vi "Inverse_Kinematics_noErrMsg_v1.vi"(4 "B3":dbl[](array[numeric]), 5 "px":dbl, 6 "pz":dbl, 7 "B2":dbl[](array[numeric]), 8 "py":dbl, 9 "B1":dbl[](array[numeric])) -> (1 "theta 3":sgl, 2 "theta 2":sgl, 3 "theta 1":sgl)   [LabVIEW 2010]
doc: "This VI converts the desired tool tip position (px,py,pz) into joint motions of theta 1, theta 2, and theta 3.\nB1, B2, and B3 are 2-element arrays containing lower and upper bounds for joint motions.\n\"Reset Inputs\" sends out a boolean value (T) if an error occurs."
panel:
  out "theta 3 LB":dbl
  out "theta 3 UB":dbl
  out "theta 2 LB":dbl
  out "theta 2 UB":dbl
  out "theta 1 LB":dbl
  out "theta 1 UB":dbl
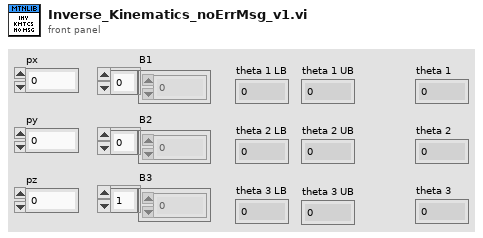
[diagram p1: front panel]
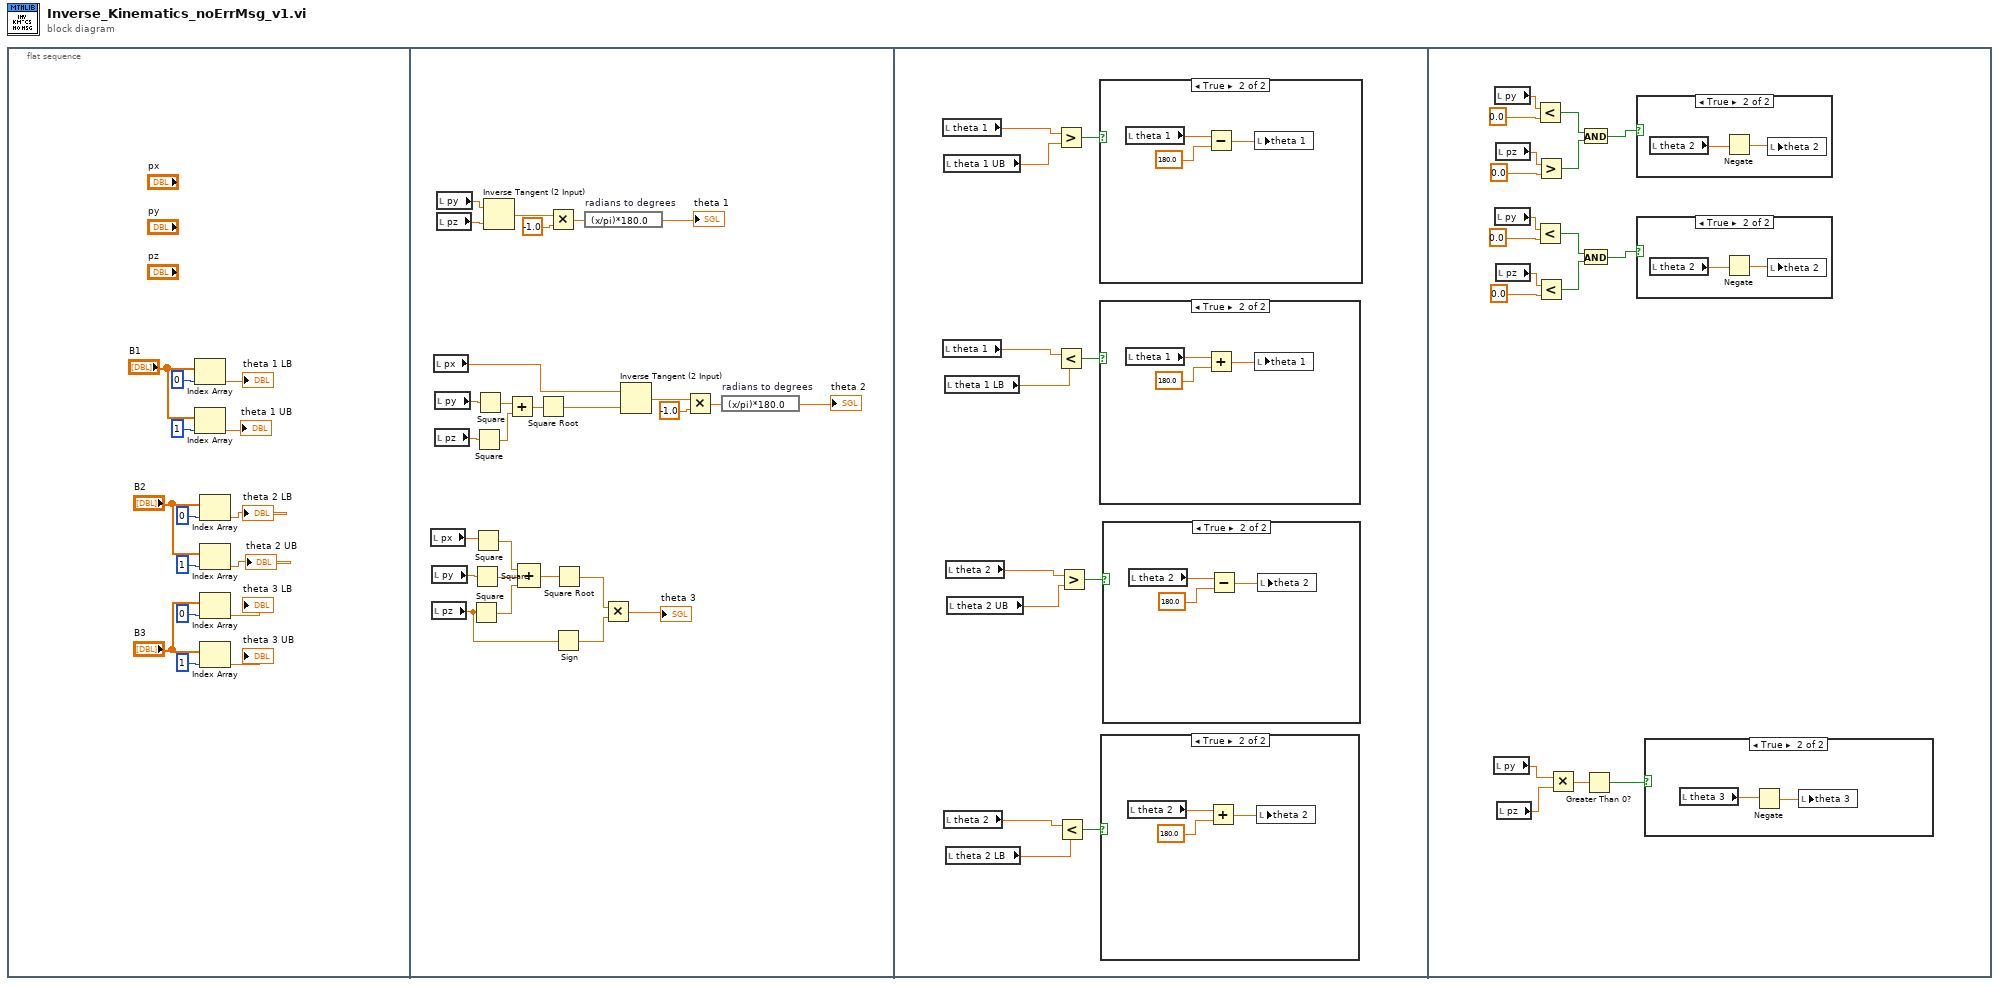
[diagram p0: block diagram]
diagram:
  n1 = flat-sequence {
    frame #0 {
      n2 = Index Array(array="B1", index=0) -> (element=→"theta 1 LB":dbl)
      n3 = Index Array(array="B1", index=1) -> (element=→"theta 1 UB":dbl)
      n4 = Index Array(array="B2", index=0) -> (element=→"theta 2 LB":dbl)
      n5 = Index Array(array="B2", index=1) -> (element=→"theta 2 UB":dbl)
      n6 = Index Array(array="B3", index=0) -> (element=→"theta 3 LB":dbl)
      n7 = Index Array(array="B3", index=1) -> (element=→"theta 3 UB":dbl)
    }
    frame #1 {
      n8 = local read "px"() -> (w38:dbl)
      n9 = local read "py"() -> (w37:dbl)
      n10 = local read "pz"() -> (w19:dbl)
      n11 = local read "px"() -> (w30:dbl)
      n12 = local read "py"() -> (w31:dbl)
      n13 = local read "pz"() -> (w32:dbl)
      n14 = local read "py"() -> (w20:dbl)
      n15 = local read "pz"() -> (w21:dbl)
      n16 = Square(x=w19) -> (x^2=w41:dbl)
      n17 = Square(x=w37) -> (x^2=w40:dbl)
      n18 = Square(x=w38) -> (x^2=w39:dbl)
      n19 = Square(x=w32) -> (x^2=w34:dbl)
      n20 = Square(x=w31) -> (x^2=w33:dbl)
      n21 = Inverse Tangent (2 Input)(1:w21, 2:w20) -> (0:w22:dbl)
      n22 = Add(x=w33, y=w34) -> (x+y=w35:dbl)
      n23 = Compound Arithmetic op=ADD(w39, w40, w41) -> (w42:dbl)
      n24 = Square Root(x=w35) -> (sqrt(x)=w36:dbl)
      n25 = Multiply(x=w22, y=sgl -1.0) -> (x*y=w24:dbl)
      n26 = Sign(1:w19) -> (0:w17:dbl)
      n27 = Square Root(x=w42) -> (sqrt(x)=w18:dbl)
      n28 = expression code="(x/pi)*180.0" "radians to degrees"(w24) -> (→"theta 1":dbl)
      n29 = Multiply(x=w18, y=w17) -> (x*y=→"theta 3":dbl)
      n30 = Inverse Tangent (2 Input)(1:w36, 2:w30) -> (0:w29:dbl)
      n31 = Multiply(x=w29, y=sgl -1.0) -> (x*y=w27:dbl)
      n32 = expression code="(x/pi)*180.0" "radians to degrees"(w27) -> (→"theta 2":dbl)
    }
    frame #2 {
      n33 = local read "theta 1"() -> (w44:sgl)
      n34 = local read "theta 1"() -> (w47:sgl)
      n35 = local read "theta 1 UB"() -> (w45:dbl)
      n36 = local read "theta 2"() -> (w50:sgl)
      n37 = local read "theta 1 LB"() -> (w46:dbl)
      n38 = local read "theta 2"() -> (w53:sgl)
      n39 = local read "theta 2 LB"() -> (w51:dbl)
      n40 = local read "theta 2 UB"() -> (w52:dbl)
      n41 = Greater?(x=w44, y=w45) -> (0:w43:bool)
      n42 = Less?(x=w47, y=w46) -> (x < y?=w48:bool)
      n43 = Less?(x=w50, y=w51) -> (x < y?=w49:bool)
      n44 = Greater?(x=w53, y=w52) -> (0:w54:bool)
      n45 = case shown="True" w43 {
        frame False {
        }
        frame True {
          n46 = local read "theta 1"() -> (w66:sgl)
          n47 = Subtract(x=w66, y=sgl 180.0) -> (x-y=w64:sgl)
          n48 = local write "theta 1"(w64) -> ()
        }
      }
      n49 = case shown="True" w48 {
        frame False {
        }
        frame True {
          n50 = local read "theta 1"() -> (w63:sgl)
          n51 = Add(x=w63, y=sgl 180.0) -> (x+y=w61:sgl)
          n52 = local write "theta 1"(w61) -> ()
        }
      }
      n53 = case shown="True" w49 {
        frame False {
        }
        frame True {
          n54 = local read "theta 2"() -> (w57:sgl)
          n55 = Add(x=w57, y=sgl 180.0) -> (x+y=w55:sgl)
          n56 = local write "theta 2"(w55) -> ()
        }
      }
      n57 = case shown="True" w54 {
        frame False {
        }
        frame True {
          n58 = local read "theta 2"() -> (w60:sgl)
          n59 = Subtract(x=w60, y=sgl 180.0) -> (x-y=w58:sgl)
          n60 = local write "theta 2"(w58) -> ()
        }
      }
    }
    frame #3 {
      n61 = local read "py"() -> (w70:dbl)
      n62 = local read "py"() -> (w83:dbl)
      n63 = local read "py"() -> (w72:dbl)
      n64 = local read "pz"() -> (w82:dbl)
      n65 = local read "pz"() -> (w73:dbl)
      n66 = local read "pz"() -> (w69:dbl)
      n67 = Less?(x=w83, y=0.0) -> (x < y?=w80:bool)
      n68 = Less?(x=w72, y=0.0) -> (x < y?=w75:bool)
      n69 = Greater?(x=w82, y=0.0) -> (0:w79:bool)
      n70 = Less?(x=w73, y=0.0) -> (x < y?=w76:bool)
      n71 = Multiply(x=w70, y=w69) -> (x*y=w68:dbl)
      n72 = And(x=w80, y=w79) -> (x .and. y?=w78:bool)
      n73 = And(x=w75, y=w76) -> (x .and. y?=w77:bool)
      n74 = Greater Than 0?(x=w68) -> (x > 0?=w67:bool)
      n75 = case shown="True" w78 {
        frame False {
        }
        frame True {
          n76 = local read "theta 2"() -> (w90:sgl)
          n77 = Negate(x=w90) -> (-x=w89:sgl)
          n78 = local write "theta 2"(w89) -> ()
        }
      }
      n79 = case shown="True" w77 {
        frame False {
        }
        frame True {
          n80 = local read "theta 2"() -> (w88:sgl)
          n81 = Negate(x=w88) -> (-x=w87:sgl)
          n82 = local write "theta 2"(w87) -> ()
        }
      }
      n83 = case shown="True" w67 {
        frame False {
        }
        frame True {
          n84 = local read "theta 3"() -> (w86:sgl)
          n85 = Negate(x=w86) -> (-x=w85:sgl)
          n86 = local write "theta 3"(w85) -> ()
        }
      }
    }
  }
